vi "read.vi"(8 "error in (no error)":errorcluster, 11 "Packet in":refnum<class "RPCFunction.lvclass">) -> (0 "error out":errorcluster, 2 "Output":string, 3 "Packet out":refnum<class "RPCFunction.lvclass">)   [LabVIEW 2011, in "mbed_LVLibrary.lvlib" / "RPCFunction.lvclass"]
uses:
  RPCFunction.lvclass
  RPCFunction.lvclass/RPCFunction.ctl
  Transport Mechanisms/mbed/mbed.lvclass
panel:
  # "The output from the mbed function"
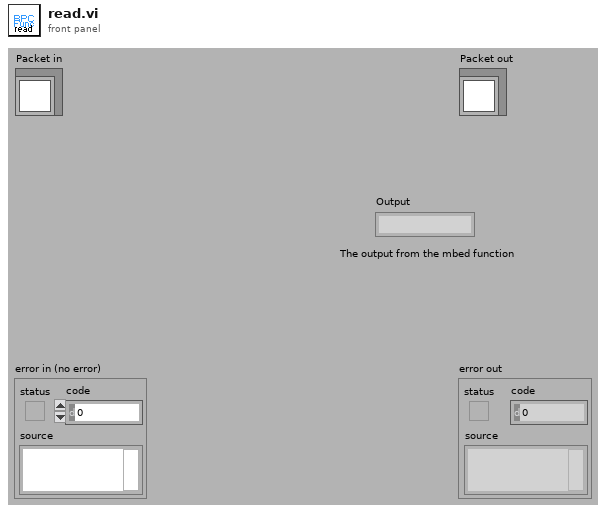
[diagram p1: front panel]
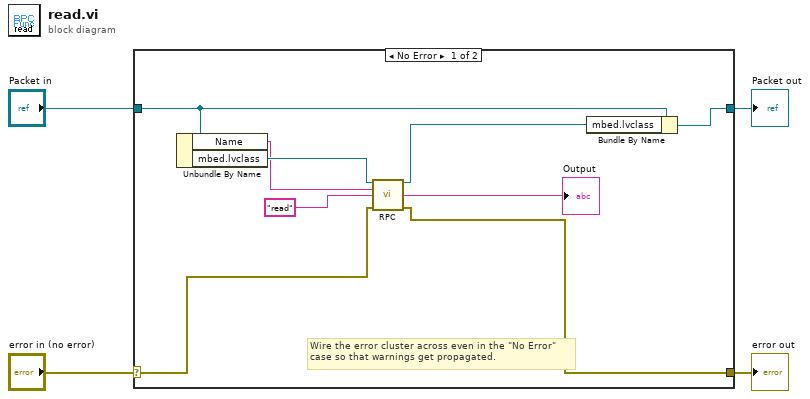
[diagram p0: block diagram]
diagram:
  n1 = case shown="No Error" "error in (no error)" {
    selector: "error in (no error)" -> [w6 w15]
    tunnel: [w5 w15] -> w3
    tunnel: [w12 w14] -> w1
    tunnel: "Packet in" -> [w13 w14]
    frame No Error {
      # "Wire the error cluster across even in the \"No Error\"\ncase so that warnings get propagated."
      n2 = Unbundle By Name(w13) -> ("Name"=w10:string, "mbed.lvclass"=w11:refnum<class "mbed.lvclass">)
      n3 = call-dynamic "RPC.vi"("mbed in"=w11, "Name"=w10, "method"="read", "error in (no error)"=w6) -> ("mbed out"=w9:refnum<class "mbed.lvclass">, "RPC Result"=→"Output":string, "error out"=w5:errorcluster)  [unwired: 9 in]
      n4 = Bundle By Name(cluster=w13, "mbed.lvclass"=w9) -> (w12:refnum<class "RPCFunction.lvclass">)
    }
    frame Error {
    }
  }
  "error out" <- w3
  "Packet out" <- w1
